vi "ma_SML Peak-hold Averaging (real input, scalar).vi"(0 "x":dbl format="%.2f", 1 "reset?":bool) -> (2 "y":dbl format="%.2f", 3 "averages sofar":dbl, 4 "data ready?":bool)   [LabVIEW 2020, in "NI_MAPro.lvlib"]
uses:
  NI_MAPro.lvlib
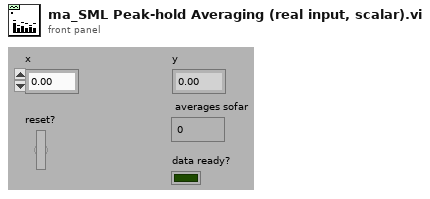
[diagram p1: front panel]
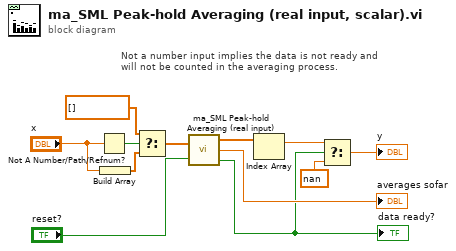
[diagram p0: block diagram]
diagram:
  # "Not a number input implies the data is not ready and \nwill not be counted in the averaging process."
  n1 = Not A Number/Path/Refnum?(number/path/refnum="x") -> (NaN/Path/Refnum?=w12:bool)
  n2 = Build Array("x") -> (w8:dbl[])
  n3 = Select(t=dbl[] [] ("x"), s=w12, f=w8) -> (s? t:f=w7:dbl[])
  n4 = call "ma_SML Peak-hold Averaging (real input).vi"("x"=w7, "reset?"="reset?") -> ("y"=w6:dbl[], "averages sofar"=→"averages sofar":dbl, "data ready?"=w4:bool)
  "data ready?" <- w4
  n5 = Index Array(array=w6) -> (element=w3:dbl)  [unwired: 1 in]
  n6 = Select(t=w3, s=w4, f=nan) -> (s? t:f=→"y":dbl)
